vi "niScope Get Stream Endpoint Handle.vi"(0 "instrument handle":refnum<k15>, 5 "stream endpoint":string="0", 11 "error in":errorcluster) -> (4 "instrument handle out":refnum<k15>, 6 "writer handle":refnum<k20>, 15 "error out":errorcluster)   [LabVIEW 2011]
doc: "Returns a writer endpoint that can be used with NI-P2P to configure a peer-to-peer stream with a digitizer endpoint."
uses:
  niScope_32.dll
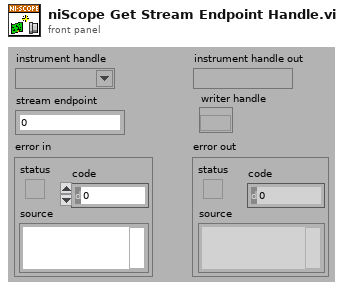
[diagram p1: front panel]
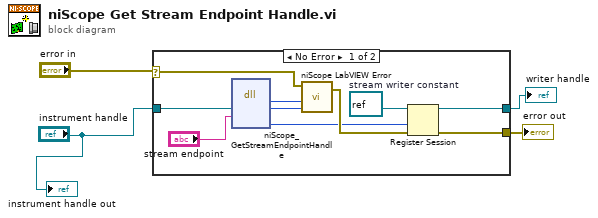
[diagram p0: block diagram]
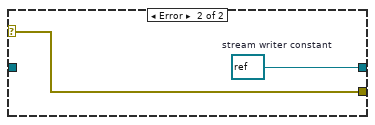
[diagram p2: hidden frame]
diagram:
  n1 = case shown="No Error" "error in" {
    selector: "error in" -> [w14 w16]
    tunnel: [w9 w16] -> w3
    tunnel: "instrument handle" -> [w13 _]
    tunnel: [w7 w15] -> w1
    frame No Error {
      w6 = refnum<k20> refnum  # stream writer constant
      n2 = dll-call lib="niScope_*.*" fn="niScope_GetStreamEndpointHandle"("instrument handle"=w13, "streamEndpoint"="stream endpoint") -> ("status"=w11:i32, "instrument handle"=w12:u32, "writerHandle"=w5:u32)  [unwired: 5 in, 2 out]
      n3 = call <instrlib>:"niScope LabVIEW Error.vi"("instrument handle"=w12, "niScope error code (0)"=w11, "error in (no error)"=w14) -> ("error out"=w10:errorcluster)  [unwired: 2 out]
      n4 = Register Session(8:w10, 9:w5, 11:w6) -> (0:w9:errorcluster, 3:w7:refnum<k20>)  [unwired: 2 in]
    }
    frame Error {
      w15 = refnum<k20> refnum  # stream writer constant
    }
  }
  "error out" <- w3
  "writer handle" <- w1
  "instrument handle out" <- "instrument handle"
